vi "Task Init.vi"(8 "error in (no error)":errorcluster, 11 "AbortManager in":refnum<class "AbortManager.lvclass">) -> (0 "error out":errorcluster, 3 "AbortManager out":refnum<class "AbortManager.lvclass">)   [LabVIEW 2020, in "Volatus.lvlib" / "AbortManager.lvclass"]
uses:
  AbortManager.lvclass
  AbortManager.lvclass/AbortManager.ctl
  Task/Task.lvclass
  lv-cdm/CDM-Config/Config Element/Config Element.lvclass
  C:/dev/lv20CE/relink/lv-volatus/Volatus/Task/Task.lvclass
  C:/Program Files (x86)/National Instruments/LabVIEW 2020/vi.lib/ActorFramework/Actor/Actor.lvclass
  C:/dev/lv20CE/relink/lv-volatus/Volatus/TaskStateHandler/TaskStateHandler.lvclass
  C:/dev/lv20CE/relink/lv-volatus/Volatus/VectoMessageHandler/VectoMessageHandler.lvclass
  C:/dev/lv20CE/relink/lv-volatus/Volatus/AbortManager/AbortManager.lvclass
  C:/dev/lv20CE/relink/lv-volatus/Volatus/Abortable/Abortable.lvclass
  C:/dev/lv20CE/relink/lv-volatus/Volatus/API Provider/API Provider.lvclass
  VolatusConfig/VolatusConfigElement/VolatusConfigElement.lvclass
  VolatusConfig/Task/Task.lvclass
  C:/dev/lv20CE/relink/lv-volatus/VolatusConfig/VolatusConfigElement/VolatusConfigElement.lvclass
  C:/dev/lv20CE/relink/lv-volatus/VolatusConfig/Task/Task.lvclass
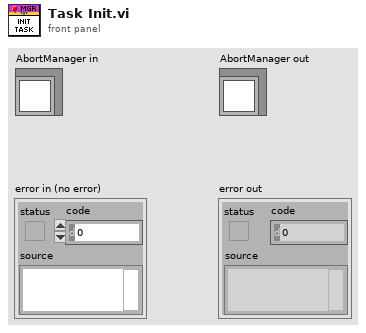
[diagram p1: front panel]
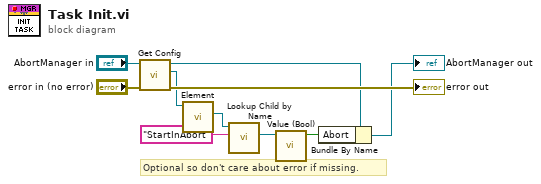
[diagram p0: block diagram]
diagram:
  # "Optional so don't care about error if missing."
  n1 = call "Get Config.vi"("error in (no error)"="error in (no error)", "Task in"="AbortManager in") -> ("error out"=→"error out":errorcluster, "Config"=w7:refnum<class "Task.lvclass">, "Task out"=w2:refnum<class "AbortManager.lvclass">)  [unwired: 7 in]
  n2 = call "Element.vi"("VolatusConfigElement in"=w7) -> ("Element"=w6:refnum<class "Config Element.lvclass">)  [unwired: 9 in, 1 out]
  n3 = call "Lookup Child by Name.vi"("Name"="StartInAbort", "Config Element in"=w6) -> ("Child"=w4:refnum<class "Config Element.lvclass">)  [unwired: 6 in, 3 out]
  n4 = call "Value (Bool).vi"("Config Element in"=w4) -> ("Bool Value"=w3:bool)  [unwired: 9 in, 1 out]
  n5 = Bundle By Name(cluster=w2, "Abort"=w3) -> (→"AbortManager out":refnum<class "AbortManager.lvclass">)
